vi "Save Cine from RAM.vi"() -> ()   [LabVIEW 2013]
doc: "This example VI demonstrates the saving of captured images stored in the internal RAM of a Phantom Camera using the Vision Research Phantom Series LabVIEW Driver."
uses:
  _Type Defs/StampTime.ctl
  _Type Defs/PhFile InfName.ctl
  VRI.lvlib
panel:
  out "Progress":u8(slide) max=100 scale=0.0..100.0
  out "Continue":bool
  out "Success":bool
  in  "Save":bool
  in  "Cine Number":u32=1 max=1
  out "Error Out":errorcluster
  in  "StampTime":T1
  in  "Camera Number":u32
  in  "error in (no error)":errorcluster
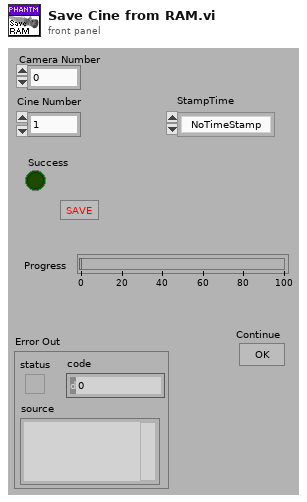
[diagram p1: front panel]
types:
  T1 = typedef "VRI.lvlib/StampTime.ctl" = enum32{"NoTimeStamp", "Time stamp", "", "Time stamp from trigger"}
  T2 = typedef "VRI.lvlib/PhFile InfName.ctl" = u32
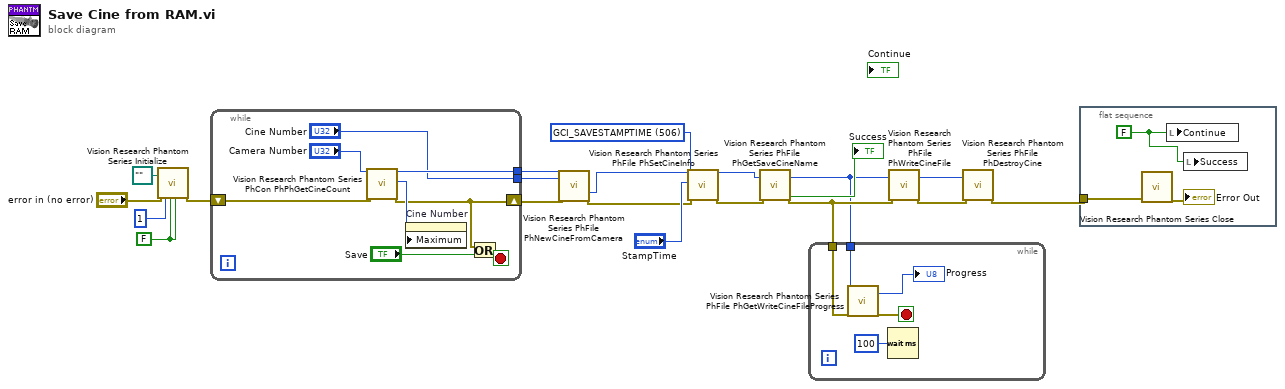
[diagram p0: block diagram]
diagram:
  w13 = T2 506 items=["GCI_CFA"=0, "GCI_FRAMERATE"=1, "GCI_EXPOSURE"=2, "GCI_AUTOEXPOSURE"=3, "GCI_REALBPP"=4, "GCI_CAMERASERIAL"=5, "GCI_HEADSERIAL0"=6, "GCI_HEADSERIAL1"=7, "GCI_HEADSERIAL2"=8, "GCI_HEADSERIAL3"=9, "GCI_TRIGTIMESEC"=10, "GCI_TRIGTIMEFR"=11, "GCI_ISFILECINE"=12, "GCI_IS16BPPCINE"=13, "GCI_ISCOLORCINE"=14, "GCI_ISMULTIHEADCINE"=15, "GCI_EXPOSURENS"=16, "GCI_EDREXPOSURENS"=17, "GCI_FRAMEDELAYNS"=19, "GCI_FROMFILETYPE"=20, "GCI_COMPRESSION"=21, "GCI_CAMERAVERSION"=22, "GCI_ROTATE"=23, "GCI_IMWIDTH"=24, "GCI_IMHEIGHT"=25, "GCI_IMWIDTHACQ"=26, "GCI_IMHEIGHTACQ"=27, "GCI_POSTTRIGGER"=28, "GCI_IMAGECOUNT"=29, "GCI_TOTALIMAGECOUNT"=30, "GCI_TRIGFRAME"=31, "GCI_AUTOEXPLEVEL"=32, "GCI_AUTOEXPTOP"=33, "GCI_AUTOEXPLEFT"=34, "GCI_AUTOEXPBOTTOM"=35, "GCI_AUTOEXPRIGHT"=36, "GCI_RECORDINGTIMEZONE"=37, "GCI_FIRSTIMAGENO"=38, "GCI_FIRSTMOVIEIMAGE"=39, "GCI_CINENAME"=40, "GCI_FRPSTEPS"=100, "GCI_FRP1X"=101, "GCI_FRP1Y"=102, "GCI_FRP2X"=103, "GCI_FRP2Y"=104, "GCI_FRP3X"=105, "GCI_FRP3Y"=106, "GCI_FRP4X"=107, "GCI_FRP4Y"=108, "GCI_WRITEERR"=109, "GCI_LENSDESCRIPTION"=110, "GCI_LENSAPERATURE"=111, "GCI_LENSFOCALLENGTH"=112, "GCI_WB"=200, "GCI_WBVIEW"=201, "GCI_BRIGHT"=202, "GCI_CONTRAST"=203, "GCI_GAMMA"=204, "GCI_GAMMAR"=223, "GCI_GAMMAB"=224, "GCI_SATURATION"=205, "GCI_HUE"=206, "GCI_FLIPH"=207, "GCI_FLIPV"=208, "GCI_FILTERCODE"=209, "GCI_IMFILTER"=210, "GCI_INTALGO"=211, "GCI_PEDESTALR"=212, "GCI_PEDESTALG"=213, "GCI_PEDESTALB"=214, "GCI_FLARE"=225, "GCI_CHROMA"=226, "GCI_TONE"=227, "GCI_ENABLEMATRICES"=228, "GCI_USERMATRIX"=229, "GCI_RESAMPLEACTIVE"=215, "GCI_RESAMPLEWIDTH"=216, "GCI_RESAMPLEHEIGHT"=217, "GCI_CROPACTIVE"=218, "GCI_CROPRECTANGLE"=219, "GCI_OFFSET16_8"=220, "GCI_GAIN16_8"=221, "GCI_DEMOSAICINGFUNCPTR"=222, "GCI_VFLIPVIEWACTIVE"=300, "GCI_MAXIMGSIZE"=400, "GCI_FRPIMGNOARRAY"=450, "GCI_FRPRATEARRAY"=451, "GCI_FRPSHAPEARRAY"=452, "GCI_TRIGTC"=470, "GCI_TRIGTCU"=471, "GCI_PBRATE"=472, "GCI_TCRATE"=473, "GCI_SAVERANGE"=500, "GCI_SAVEFILENAME"=501, "GCI_SAVEFILETYPE"=502, "GCI_SAVE16BIT"=503, "GCI_SAVEPACKED"=504, "GCI_SAVEXML"=505, "GCI_SAVESTAMPTIME"=506, "GCI_SAVEAVIFRAMERATE"=520, "GCI_SAVEAVICOMPRESSORLIST"=521, "GCI_SAVEAVICOMPRESSORINDEX"=522, "GCI_SAVEDPXLSB"=530, "GCI_SAVEDPXTO10BPS"=531, "GCI_SAVEDPXDATAPACKING"=532, "GCI_SAVEDPX10BITLOG"=533, "GCI_SAVEDPXEXPORTLOGLUT"=534, "GCI_SAVEDPX10BITLOGREFWHITE"=535, "GCI_SAVEDPX10BITLOGREFBLACK"=536, "GCI_SAVEDPX10BITLOGGAMMA"=537, "GCI_SAVEDPX10BITLOGFILMGAMMA"=538, "GCI_SAVEQTPLAYBACKRATE"=550, "GCI_SAVECCIQUALITY"=560, "GCI_UNCALIBRATEDIMAGE"=600, "GCI_NOPROCESSING"=601, "GCI_BADPIXELREPAIR"=602] ("InfName [in]")
  w17 = FALSE ("ID Query (T: Check)")
  n1 = call "Vision Research Phantom Series Initialize.vi"("Storage Path (\"\")"=path "" ("Storage Path (\"\")"), "error in (no error)"="error in (no error)", "CallID"=u32 1, "ID Query (T: Check)"=w17, "Reset (F: Don't Reset)"=w17) -> ("Error Out"=w14:errorcluster)  [unwired: 14 out]
  n2 = while {
    tunnel: [w28] -> w20
    tunnel: ["Cine Number"] -> w19
    shift-right: [w21] -> w10
    shift-left: w14 -> [w26]
    stop <- w22 stop-if-true
    n3 = call "Vision Research Phantom Series PhCon PhPhGetCineCount.vi"("CN in"="Camera Number", "Error In (no error)"=w26) -> ("CN out"=w28:u32, "pRAMCount"=w24:u32, "Error Out"=w21:errorcluster)  [unwired: 15 out]
    n4 = property on="Cine Number" class="DigNum (strict)"("Maximum"=w24) -> ()  [unwired: 2 in, 2 out]
    n5 = Or(x=w21, y="Save") -> (x .or. y?=w22:bool)
  }
  n6 = call "Vision Research Phantom Series PhFile PhNewCineFromCamera.vi"("Camera Number in"=w20, "CineNr in"=w19, "Error In (no error)"=w10) -> ("pCH"=w5:u32, "Error Out"=w4:errorcluster)  [unwired: 1 in, 14 out]
  n7 = call "Vision Research Phantom Series PhFile PhSetCineInfo.vi"("CH [in]"=w5, "InfName [in]"=w13, "pInfVal [in]"="StampTime", "Error In (no error)"=w4) -> ("CH [out]"=w8:u32, "Error Out"=w9:errorcluster)  [unwired: 14 out]
  n8 = call "Vision Research Phantom Series PhFile PhGetSaveCineName.vi"("CH in"=w8, "Error In (no error)"=w9) -> ("CH out"=w6:u32, "Success"=→"Success":bool, "Error Out"=w7:errorcluster)  [unwired: 15 out]
  n9 = while {
    tunnel: w7 -> [w33]
    tunnel: w6 -> [w32]
    stop <- w29 stop-if-true
    n10 = call "Vision Research Phantom Series PhFile PhGetWriteCineFileProgress.vi"("CH [in]"=w32, "Error In (no error)"=w33) -> ("pProgressPercent [out]"=→"Progress":u32, "Error Out"=w29:errorcluster)  [unwired: 16 out]
    n11 = Wait (ms)(milliseconds to wait=u32 100) -> ()  [unwired: 1 out]
  }
  n12 = call "Vision Research Phantom Series PhFile PhWriteCineFile.vi"("CH in"=w6, "Error In (no error)"=w7) -> ("CH out"=w1:u32, "Error Out"=w3:errorcluster)  [unwired: 1 in, 15 out]
  n13 = call "Vision Research Phantom Series PhFile PhDestroyCine.vi"("CH in"=w1, "Error In (no error)"=w3) -> ("Error Out"=w2:errorcluster)  [unwired: 17 out]
  n14 = flat-sequence {
    tunnel: w2 -> [w35]
    frame #0 {
      w34 = FALSE
      n15 = call "Vision Research Phantom Series Close.vi"("Error In (no error)"=w35) -> ("Error Out"=→"Error Out":errorcluster)  [unwired: 18 out]
      n16 = local write "Continue"(w34) -> ()
      n17 = local write "Success"(w34) -> ()
    }
  }
